vi "Corrected current calculator (SubVI).vi"(9 "Necessary current":dbl, 10 "I_set old":dbl, 11 "Actual current":dbl) -> (3 "I_set new":dbl)   [LabVIEW 2018]
panel:
  # "This subVI calculates the \"mistake\" in the current flowing through the coils, and then calculates the new I that should be set to the power supply."
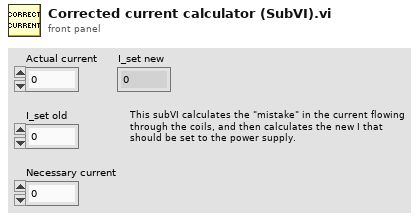
[diagram p1: front panel]
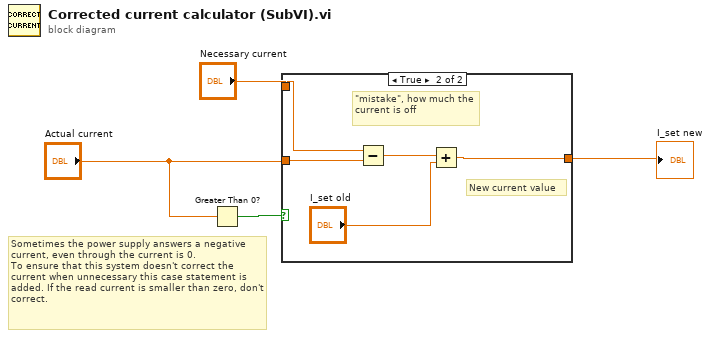
[diagram p0: block diagram]
diagram:
  # "Sometimes the power supply answers a negative current, even through the current is 0. \nTo ensure that this system doesn't correct the current when unnecessary this case statement is added. If the read current is smaller than zero, don't correct."
  n1 = Greater Than 0?(x="Actual current") -> (x > 0?=w1:bool)
  n2 = case shown="True" w1 {
    tunnel: [w5 w10] -> w4
    tunnel: "Actual current" -> [_ w8]
    tunnel: "Necessary current" -> [w5 w7]
    frame False {
    }
    frame True {
      # "New current value"
      # "\"mistake\", how much the current is off"
      n3 = Subtract(x=w7, y=w8) -> (x-y=w9:dbl)
      n4 = Add(x=w9, y="I_set old") -> (x+y=w10:dbl)
    }
  }
  "I_set new" <- w4
